vi "Forward Direct Message.vi"(8 "error in (no error)":errorcluster, 10 "Message":T1, 11 "Chat Window Model in":refnum<class "Chat Window Model.lvclass">) -> (0 "error out":errorcluster, 3 "Chat Window Model out":refnum<class "Chat Window Model.lvclass">)   [LabVIEW 2019, in "Chat Window Model.lvlib" / "Chat Window Model.lvclass"]
uses:
  Chat Window Model.lvclass
  C:/Program Files/National Instruments/LabVIEW 2019/vi.lib/ActorFramework/Actor/Actor.lvclass
  Controls/Message Control.ctl
  <vilib>/ActorFramework/Actor/Actor.lvclass/Actor.ctl
  <vilib>/ActorFramework/Message Enqueuer/Message Enqueuer.lvclass/Message Enqueuer.ctl
  Chat Window Model.lvclass/Chat Window Model.ctl
  Chat Window Model Messages/Preserve Sent Message Msg/Preserve Sent Message Msg.lvclass/Preserve Sent Message Msg.ctl
  Chat Window Model Messages/Direct Message Sent Msg/Direct Message Sent Msg.lvclass/Direct Message Sent Msg.ctl
  <vilib>/ActorFramework/Message Enqueuer/Init from Existing Queue.vi
  <vilib>/ActorFramework/Message Enqueuer/Enqueue.vi
  Chat Window Model Messages/Preserve Sent Message Msg/Preserve Sent Message Msg.lvclass
  C:/Program Files/National Instruments/LabVIEW 2019/vi.lib/ActorFramework/Message/Message.lvclass
  Chat Window Model Messages/Direct Message Sent Msg/Direct Message Sent Msg.lvclass
  <vilib>/ActorFramework/Message Priority Queue/Priority Enqueue.vi
  <vilib>/ActorFramework/Message Enqueuer/Message Enqueuer.lvclass
  <vilib>/ActorFramework/Actor/Actor.lvclass
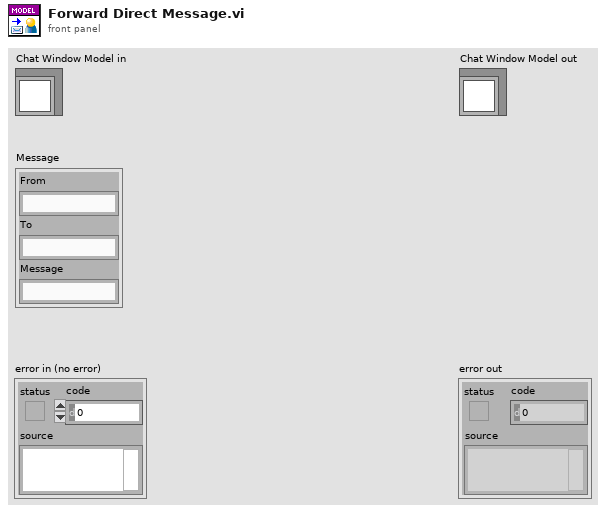
[diagram p1: front panel]
types:
  T1 = typedef "Message Control.ctl" = cluster{"From":string, "To":string, "Message":string}
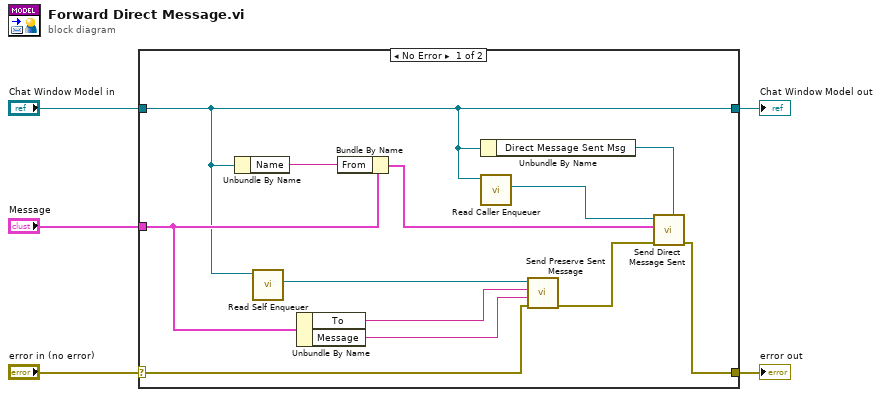
[diagram p0: block diagram]
diagram:
  n1 = case shown="No Error" "error in (no error)" {
    selector: "error in (no error)" -> [w9 w19]
    tunnel: [w15 w19] -> w4
    tunnel: [w7 w18] -> w2
    tunnel: "Chat Window Model in" -> [w7 w18]
    tunnel: "Message" -> [w12 _]
    frame No Error {
      n2 = Unbundle By Name(w7) -> ("Name"=w13:string)
      n3 = call <vilib>:"Read Self Enqueuer.vi"("Actor"=w7) -> ("Self Enqueuer"=w6:refnum<class "Message Enqueuer.lvclass">)  [unwired: 10 in]
      n4 = Unbundle By Name(w12) -> ("To"=w10:string, "Message"=w11:string)
      n5 = Bundle By Name(cluster=w12, "From"=w13) -> (w14:T1)
      n6 = Unbundle By Name(w7) -> ("Direct Message Sent Msg"=w17:refnum<class "Direct Message Sent Msg.lvclass">)
      n7 = call <vilib>:"Read Caller Enqueuer.vi"("Actor"=w7) -> ("Caller Enqueuer"=w16:refnum<class "Message Enqueuer.lvclass">)  [unwired: 10 in]
      n8 = call "Send Preserve Sent Message.vi"("error in (no error)"=w9, "Sent Message"=w11, "To"=w10, "Message Enqueuer"=w6) -> ("error out"=w8:errorcluster)  [unwired: 6 in, 1 out]
      n9 = call "Send Direct Message Sent.vi"("Message Type"=w17, "error in (no error)"=w8, "Message"=w14, "Message Enqueuer"=w16) -> ("error out"=w15:errorcluster)  [unwired: 6 in, 1 out]
    }
    frame Error {
    }
  }
  "error out" <- w4
  "Chat Window Model out" <- w2
